vi "SQL_test_data_select.vi"(11 "通道名称":string="声发射") -> (2 "error out":errorcluster, 3 "数组":dbl[][](array[numeric]))   [LabVIEW 2014]
panel:
  out "解析时间":u32
  out "查询时间":u32
  out "毫秒计时值 2":u32
  out "毫秒计时值":u32
  out "波形图":dbl[][](graph)
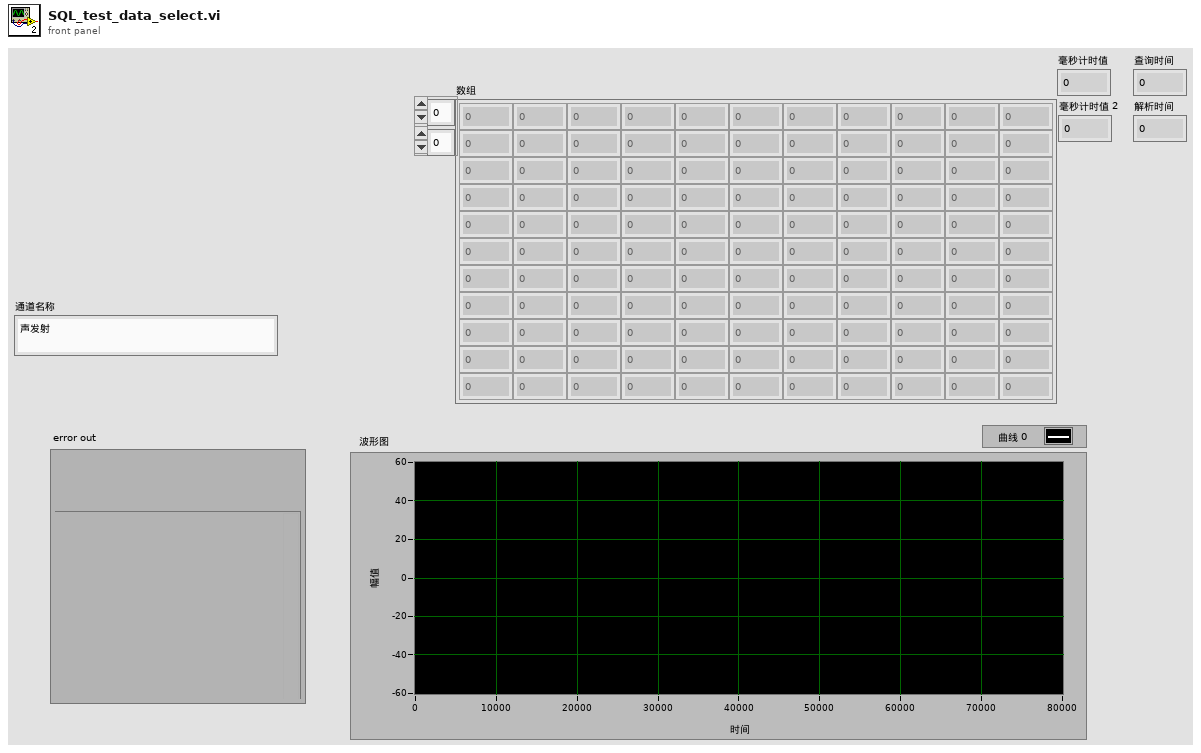
[diagram p1: front panel]
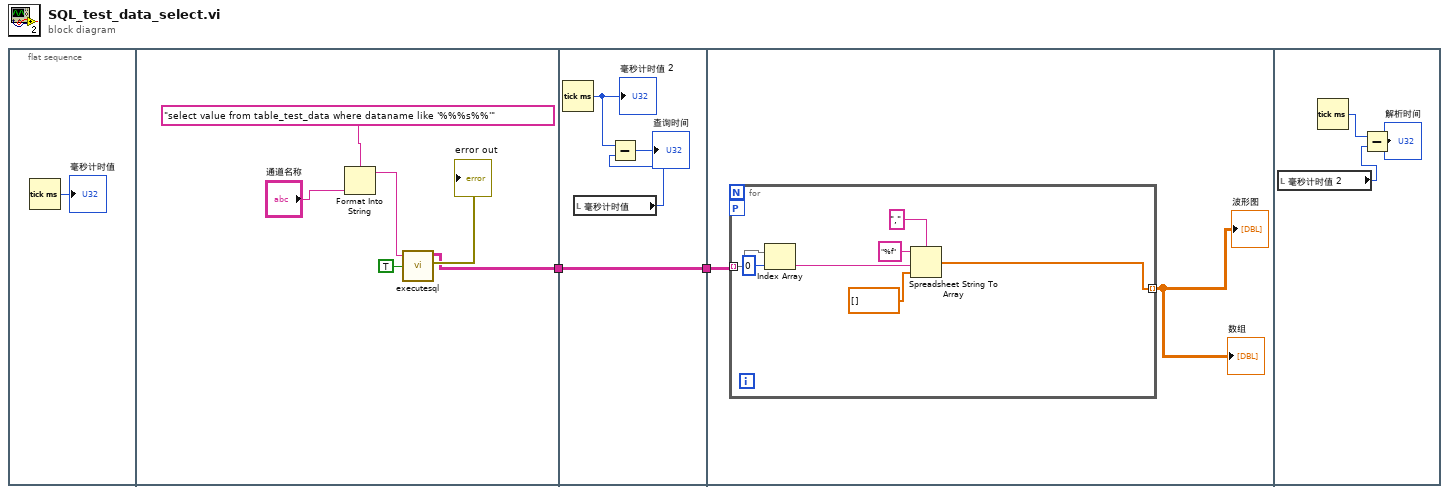
[diagram p0: block diagram]
diagram:
  n1 = flat-sequence {
    tunnel: [w4] -> w2
    tunnel: w2 -> [w13]
    tunnel: [w13] -> w1
    tunnel: w1 -> [w15]
    frame #0 {
      n2 = Tick Count (ms)() -> (millisecond timer value=→"毫秒计时值":u32)
    }
    frame #1 {
      n3 = Format Into String(format string="select value from table_test_data where dataname like '%%%s%%'", "通道名称") -> (resulting string=w7:string)  [unwired: 2 in, 1 out]
      n4 = call "executesql.vi"("Return Data (T)"=TRUE, "Command Text"=w7) -> ("error out"=→"error out":errorcluster, "Data"=w4:string[][])  [unwired: 5 in]
    }
    frame #2 {
      n5 = Tick Count (ms)() -> (millisecond timer value=w12:u32)
      "毫秒计时值 2" <- w12
      n6 = local read "毫秒计时值"() -> (w11:u32)
      n7 = Subtract(x=w12, y=w11) -> (x-y=→"查询时间":u32)
    }
    frame #3 {
      n8 = for "For循环" {
        tunnel: [w19] -> w14 mode=indexing
        tunnel: w15 -> [w22] mode=indexing
        workers-P: _ -> [_]
        n9 = Index Array(array=w22, index=0 ("索引")) -> (element=w20:string)
        n10 = Spreadsheet String To Array(delimiter (Tab)="," ("分隔符(Tab)"), format string="%f" ("格式字符串"), spreadsheet string=w20, array type (2D Dbl)=dbl[] [] ("数组类型(2D Dbl)")) -> (array=w19:dbl[])
      }
      "波形图" <- w14
      "数组" <- w14
    }
    frame #4 {
      n11 = local read "毫秒计时值 2"() -> (w24:u32)
      n12 = Tick Count (ms)() -> (millisecond timer value=w25:u32)
      n13 = Subtract(x=w25, y=w24) -> (x-y=→"解析时间":u32)
    }
  }
